vi "Read Mods.vi"(8 "error in (no error)":errorcluster, 11 "ControlMouseUpMsg in":refnum<class "ControlMouseUpMsg.lvclass">) -> (0 "error out":errorcluster, 2 "Mods":cluster{"Double Click":bool, "Menu Key":bool}, 3 "ControlMouseUpMsg out":refnum<class "ControlMouseUpMsg.lvclass">)   [LabVIEW 2020, in "ActorEvents.lvlib" / "ControlMouseUpMsg.lvclass"]
uses:
  <vilib>/gpm_packages/@cs/mva-viewable/Source/ActorEvents/IEventAggregator Messages/ControlMouseUpMsg/ControlMouseUpMsg.lvclass
  <vilib>/gpm_packages/@cs/mva-viewable/Source/ActorEvents/IEventAggregator Messages/ControlMouseUpMsg/ControlMouseUpMsg.lvclass/ControlMouseUpMsg.ctl
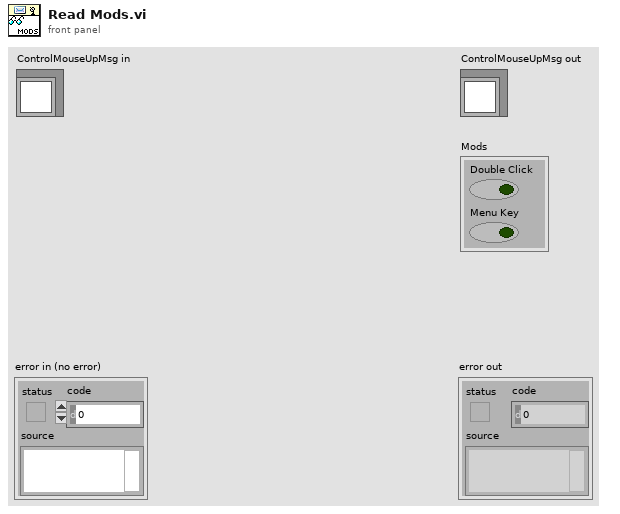
[diagram p1: front panel]
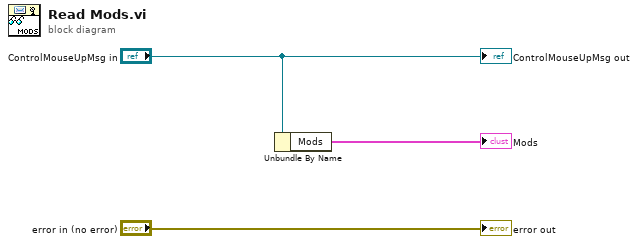
[diagram p0: block diagram]
diagram:
  n1 = Unbundle By Name("ControlMouseUpMsg in") -> ("Mods"=→"Mods":cluster{"Double Click":bool, "Menu Key":bool})
  "error out" <- "error in (no error)"
  "ControlMouseUpMsg out" <- "ControlMouseUpMsg in"
